vi "rohitwhile.vi"() -> ()   [LabVIEW 2009]
panel:
  in  "?":bool
  out "Random":dbl
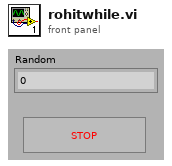
[diagram p1: front panel]
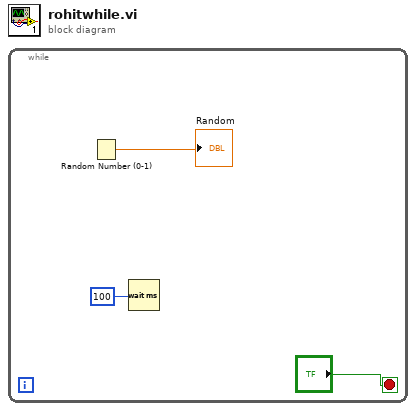
[diagram p0: block diagram]
diagram:
  n1 = while {
    stop <- "?" stop-if-true
    n2 = Random Number (0-1)() -> (number: 0 to 1=→"Random":dbl)
    n3 = Wait (ms)(milliseconds to wait=100) -> ()  [unwired: 1 out]
  }
